vi "VarNameFromMenuTag.vi"(8 "error in (no error)":errorcluster, 10 "VariableManager Ref in":refnum<vi>, 11 "Tag in":string) -> (0 "error out":errorcluster, 3 "VariableName":string)   [LabVIEW 2013]
uses:
  VariableManagerCodes/VariableManager/VariableManager.lvclass
  VariableManagerCodes/Variable/Variable.lvclass
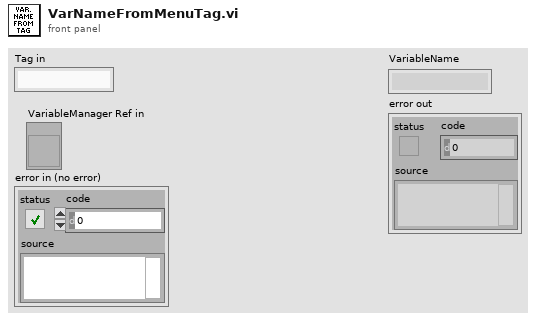
[diagram p1: front panel]
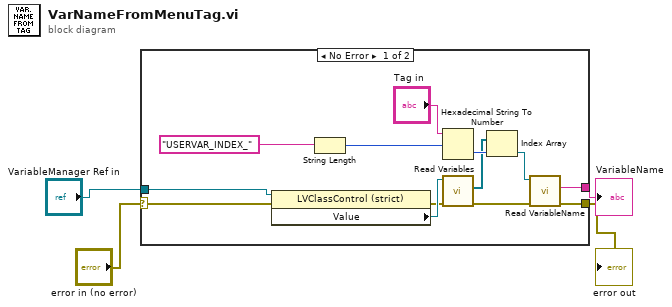
[diagram p0: block diagram]
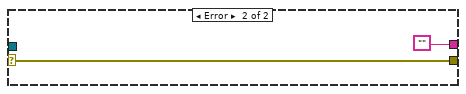
[diagram p2: hidden frame]
diagram:
  n1 = case shown="No Error" "error in (no error)" {
    selector: "error in (no error)" -> [w5 w19]
    tunnel: "VariableManager Ref in" -> [w12 _]
    tunnel: [w6 w19] -> w3
    tunnel: [w7 ""] -> w1
    frame No Error {
      n2 = property class="LVClassControl (strict)"(reference=w12, error in=w5) -> (error out=w11:errorcluster, "Value"=w13:refnum<class "VariableManager.lvclass">)  [unwired: 1 out]
      n3 = String Length(string="USERVAR_INDEX_") -> (length=w17:i32)
      n4 = Hexadecimal String To Number(string="Tag in", offset=w17) -> (number=w14:u32)  [unwired: 1 in, 1 out]
      n5 = call-dynamic "Read Variables.vi"("error in (no error)"=w11, "VariableManager in"=w13) -> ("error out"=w9:errorcluster, "Variables"=w10:refnum<class "Variable.lvclass">[])  [unwired: 7 in, 1 out]
      n6 = Index Array(array=w10, index=w14) -> (element=w8:refnum<class "Variable.lvclass">)
      n7 = call-dynamic "Read VariableName.vi"("error in (no error)"=w9, "Variable in"=w8) -> ("error out"=w6:errorcluster, "VariableName"=w7:string)  [unwired: 7 in, 1 out]
    }
    frame Error {
    }
  }
  "VariableName" <- w1
  "error out" <- w3
